vi "Document_CreateNewParagraphStyle.vi"(8 "error in":errorcluster, 10 "styleName":string, 11 "document":refnum<k24>) -> (0 "error out":errorcluster, 2 "Paragraph Style":refnum<k24>, 3 "document out":refnum<k24>)   [LabVIEW 2009]
uses:
  C:/Projets/LAVAG/OpenOfficeRGT/AODL/DLLs/AODL.dll
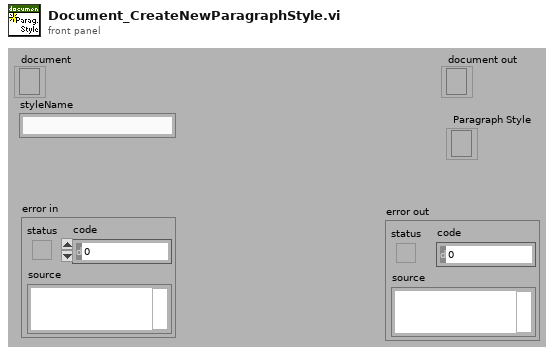
[diagram p1: front panel]
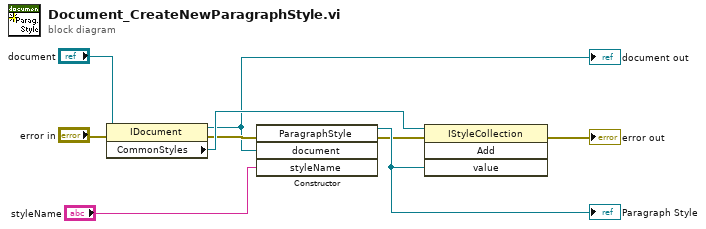
[diagram p0: block diagram]
diagram:
  n1 = property class="IDocument"(reference="document", error in="error in") -> (reference out=w1:refnum<k24>, error out=w6:errorcluster, "CommonStyles"=w8:refnum<k24>)
  "document out" <- w1
  n2 = constructor class="ParagraphStyle"(error in=w6, "document"=w1, "styleName"="styleName") -> (reference out=w7:refnum<k24>, error out=w4:errorcluster)  [unwired: 2 in, 3 out]
  "Paragraph Style" <- w7
  n3 = invoke class="IStyleCollection" method="Add"(reference=w8, error in=w4, "value"=w7) -> (error out=→"error out":errorcluster)  [unwired: 1 in, 3 out]
